vi "macro_Translation3d_X_Y_Z.vi"   [LabVIEW 2019, in "Trajectory_Library.lvlib"]
uses:
  Trajectory_Library.lvlib
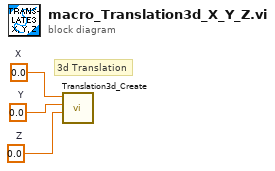
[diagram p0: block diagram]
diagram:
  w1 = 0.0  # Z
  w2 = 0.0  # X
  w3 = 0.0  # Y
  # "3d Translation"
  n1 = call "Translation3d_Create.vi"("Z"=w1, "Y"=w3, "X"=w2) -> ()  [unwired: 8 in, 1 out]
